vi "Dispose.vi"(8 "error in":errorcluster, 11 "NYStyleClamPizza":refnum<class "NYStyleClamPizza.lvclass">) -> (0 "error out":errorcluster)   [LabVIEW 2020, in "FactoryMethod.lvlib" / "PizzaFactoryMethod.lvlib" / "NYStyleClamPizza.lvclass"]
uses:
  NYStyleClamPizza.lvclass
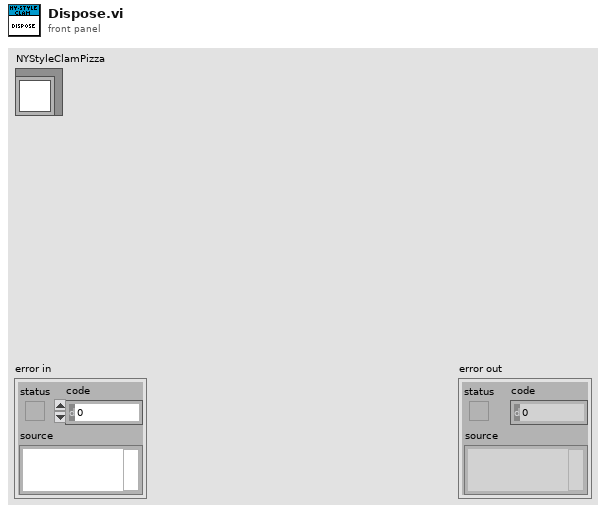
[diagram p1: front panel]
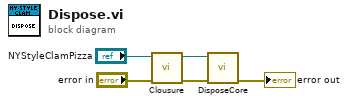
[diagram p0: block diagram]
diagram:
  n1 = call-dynamic "Clousure.vi"("error in"="error in", "NYStyleClamPizza"="NYStyleClamPizza") -> ("error out"=w3:errorcluster, "NYStyleClamPizza"=w4:refnum<class "NYStyleClamPizza.lvclass">)  [unwired: 8 in]
  n2 = call-dynamic "DisposeCore.vi"("error in (no error)"=w3, "NYStyleClamPizza"=w4) -> ("error out"=→"error out":errorcluster)  [unwired: 8 in, 1 out]
